vi "Benchmark Match Key Regex.vi"() -> ()   [LabVIEW 2019, in "Instrument.Lockin.lvlib" / "Instrument.Lockin.lvclass"]
uses:
  Instrument.Lockin.lvclass
  Typedefs/Results Type--Enum.ctl
panel:
  out "x/y":dbl format="%#_6p"
  in  "Numeric":i32
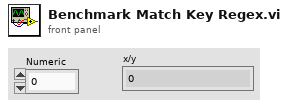
[diagram p1: front panel]
types:
  T1 = typedef "Instrument.Lockin.lvlib/Instrument.Lockin.lvclass/Results Type--Enum.ctl" = enum16{"X", "Y", "R", "Theta", "Mean"}
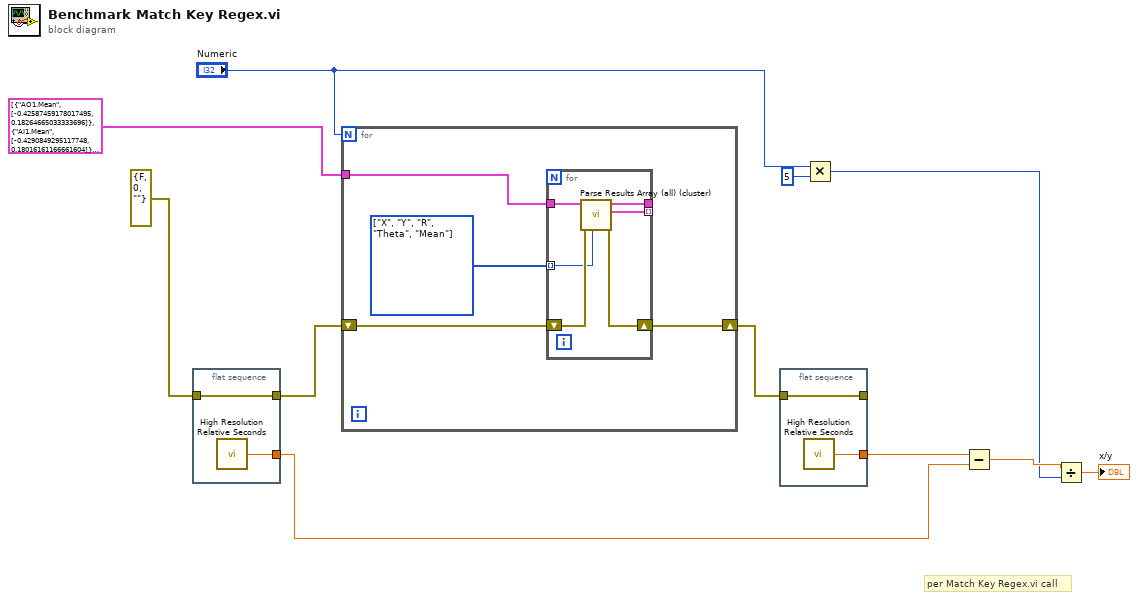
[diagram p0: block diagram]
diagram:
  # "per Match Key Regex.vi call"
  n1 = flat-sequence {
    tunnel: [w13] -> w11
    tunnel: errorcluster {"status"=FALSE, "code"=0, "source"=""} ("error in (no error)") -> [w13]
    tunnel: [w12] -> w6
    frame #0 {
      n2 = call <vilib>:"High Resolution Relative Seconds.vi"() -> ("relative seconds"=w12:dbl)
    }
  }
  n3 = for {
    N: "Numeric" -> [_]
    tunnel: cluster{"key":string, "value":dbl[]}[] [{"key"="AO1.Mean", "value"=[-0.42587459178017495, 0.18264665033333696]}, {"key"="AI1.Mean", "value"=[-0.4290849295117748, 0.18016161166661604]}, {"key"="AI2.Mean", "value"=[2.3290662181554866, 2.329061898164071]}, {"key"="AI3.Mean", "value"=[2.3286674844515876, 2.3286659984724327]}, {"key"="AI4.Mean", "value"=[2.3286165963889176, 2.3286136815976115]}, {"key"="AI1.Ref1.X", "value"=[-0.12277744185954602, -0.1254216509868524]}, {"key"="AI1.Ref1.Y", "value"=[0.7276681956673122, 0.738013976896093]}, {"key"="AI1.Ref1.R", "value"=[0.7379534559952247, 0.7485954986708474]}, {"key"="AI1.Ref1.Theta", "value"=[99.57715463025741, 99.64497239901199]}, {"key"="AI2.Ref1.X", "value"=[-0.00953516324099959, -0.025975604173804456]}, {"key"="AI2.Ref1.Y", "value"=[0.04058421084191648, 0.04510642963116445]}, {"key"="AI2.Ref1.R", "value"=[0.04168929727992115, 0.05205114798220456]}, {"key"="AI2.Ref1.Theta", "value"=[103.22170639403991, 119.93650630093333]}, {"key"="AI3.Ref1.X", "value"=[-0.00953305366895399, -0.025970726881972772]}, {"key"="AI3.Ref1.Y", "value"=[0.040577651522379896, 0.04509913577963056]}, {"key"="AI3.Ref1.R", "value"=[0.04168242933571479, 0.052042393323593186]}, {"key"="AI3.Ref1.Theta", "value"=[103.22094569305301, 119.93586044853791]}, {"key"="AI4.Ref1.X", "value"=[-0.009532969460117663, -0.025970270788949423]}, {"key"="AI4.Ref1.Y", "value"=[0.04057624545500691, 0.045097658730612576]}, {"key"="AI4.Ref1.R", "value"=[0.04168104127721026, 0.05204088573260602]}, {"key"="AI4.Ref1.Theta", "value"=[103.22127505336906, 119.93623681607122]}] ("Results (Dictionary)") -> [w14]
    shift-right: [w15] -> w9
    shift-left: w11 -> [w16]
    w17 = T1[] [enum."X", enum."Y", enum."R", enum."Theta", enum."Mean"] items=["X", "Y", "R", "Theta", "Mean"] ("Array")
    n4 = for {
      tunnel: w14 -> [w23]
      tunnel: [w21] -> _
      tunnel: w17 -> [w20] mode=indexing
      tunnel: [w18] -> _ mode=indexing
      shift-right: [w19] -> w15
      shift-left: w16 -> [w22]
      n5 = call "Parse Results Array (all) (cluster).vi"("Type"=w20, "error in (no error)"=w22, "Results (Dictionary)"=w23) -> ("error out"=w19:errorcluster, "Data"=w18:cluster{"value":dbl[]}[], "Results (Dictionary)"=w21:cluster{"key":string, "value":dbl[]}[])  [unwired: 5 in, 1 out]
    }
  }
  n6 = flat-sequence {
    tunnel: [w25] -> _
    tunnel: w9 -> [w25]
    tunnel: [w24] -> w7
    frame #0 {
      n7 = call <vilib>:"High Resolution Relative Seconds.vi"() -> ("relative seconds"=w24:dbl)
    }
  }
  n8 = Multiply(x="Numeric", y=5) -> (x*y=w1:i32)
  n9 = Subtract(x=w7, y=w6) -> (x-y=w5:dbl)
  n10 = Divide(x=w5, y=w1) -> (x/y=→"x/y":dbl)
